vi "Result_Test.vi"(8 "error in (no error)":errorcluster caption="entrée d'erreur (pas d'erreur)", 11 "Flash_Jlink en entrée":refnum<class "P2265_SwitchOff_Test.lvclass">) -> (0 "error out":errorcluster caption="sortie d'erreur", 3 "Flash_Jlink en sortie":refnum<class "P2265_SwitchOff_Test.lvclass">)   [LabVIEW 2020, in "Library Test.lvlib" / "P2265_SwitchOff_Test.lvclass"]
uses:
  P2265_SwitchOff_Test.lvclass
  C:/Users/ngarcin/OneDrive - Altyor/Standard TB/Class/Test/Test (Default)/Test (Default).lvclass
  JSON API/JSON Value/Set from JSON string.vi
  JSON API/JSON Value/JSON Value.lvclass
  Test_Wtih_Instr/Test_With_Inst.lvclass
  P2265_SwitchOff_Test.lvclass/P2265_SwitchOff_Test.ctl
  JSON API/Variant JSON/Variant JSON.lvlib
  JSON API/Get Polymorphic/JSON GetSet.lvlib
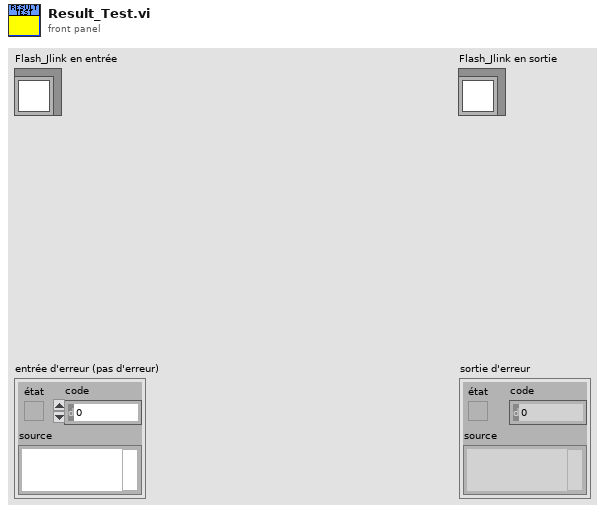
[diagram p1: front panel]
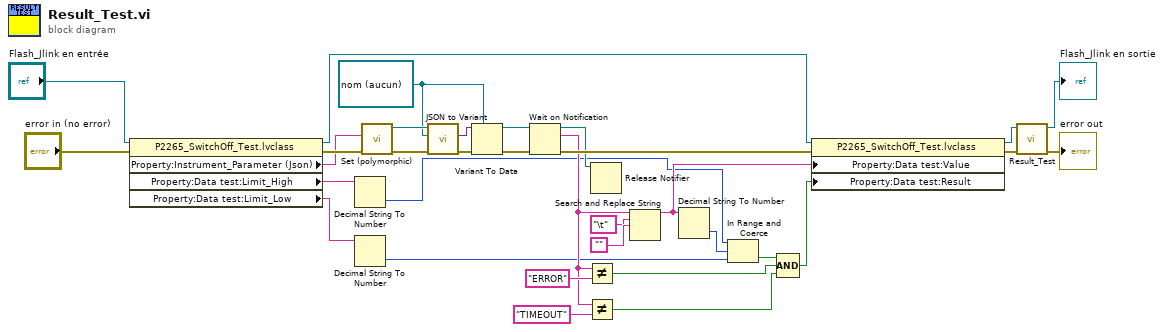
[diagram p0: block diagram]
diagram:
  w21 = refnum<notifier> refnum ("notificateur en sortie")
  n1 = property class="P2265_SwitchOff_Test.lvclass"(reference="Flash_Jlink en entrée", error in="error in (no error)") -> (reference out=w11:refnum<class "P2265_SwitchOff_Test.lvclass">, error out=w19:errorcluster, "Property:Instrument_Parameter (Json)"=w14:string, "Property:Data test:Limit_High"=w6:string, "Property:Data test:Limit_Low"=w5:string)
  n2 = Decimal String To Number(string=w6) -> (number=w4:i32)  [unwired: 2 in, 1 out]
  n3 = Decimal String To Number(string=w5) -> (number=w3:i32)  [unwired: 2 in, 1 out]
  n4 = call-poly "Set (polymorphic).vi"("error in (no error)"=w19, "JSON stream"=w14) -> ("error out"=w23:errorcluster, "JSON Value out"=w25:refnum<class "JSON Value.lvclass">)  [unwired: 7 in, 1 out]
  n5 = call "JSON to Variant.vi"("error in (no error)"=w23, "Variant (Data Type)"=w21, "JSON Value"=w25) -> ("error out"=w24:errorcluster, "Variant out"=w22:variant)  [unwired: 7 in]
  n6 = Variant To Data(error in=w24, type=w21, Variant=w22) -> (data=w17:refnum<notifier>, error out=w18:errorcluster)
  n7 = Wait on Notification(notifier=w17, error in (no error)=w18) -> (notifier out=w15:refnum<notifier>, notification=w9:string, error out=w16:errorcluster)  [unwired: 2 in, 1 out]
  n8 = Not Equal?(x=w9, y="ERROR" ("expression régulière")) -> (x != y?=w28:bool)
  n9 = Not Equal?(x=w9, y="TIMEOUT" ("expression régulière")) -> (x != y?=w27:bool)
  n10 = Release Notifier(notifier=w15) -> ()  [unwired: 2 in, 3 out]
  n11 = Search and Replace String(input string=w9, search string="\t", replace string="") -> (result string=w7:string)  [unwired: 5 in, 3 out]
  n12 = Decimal String To Number(string=w7) -> (number=w8:i32)  [unwired: 2 in, 1 out]
  n13 = In Range and Coerce(upper limit=w4, x=w8, lower limit=w3) -> (In Range?=w2:bool)  [unwired: 1 out]
  n14 = Compound Arithmetic op=AND ("Opérateur arithmétique")(w2, w28, w27) -> (w26:bool)
  n15 = property class="P2265_SwitchOff_Test.lvclass"(reference=w11, error in=w16, "Property:Data test:Value"=w7, "Property:Data test:Result"=w26) -> (reference out=w31:refnum<class "P2265_SwitchOff_Test.lvclass">, error out=w13:errorcluster)
  n16 = call-parent "Result_Test.vi"("error in (no error)"=w13, "Test_With_Inst en entrée"=w31) -> ("error out"=→"error out":errorcluster, "Test_With_Inst en sortie"=→"Flash_Jlink en sortie":refnum<class "P2265_SwitchOff_Test.lvclass">)  [unwired: 8 in]
